vi "Pose3d_New.vi"(8 "Rotation3d":T1={"Q_quaternion"={"R"=1.0, "V"=[0.0, 0.0, 0.0]}}, 9 "z":dbl, 10 "Y":dbl, 11 "X":dbl) -> (3 "out Pose3d":T3={"Translation3d"={"X"=0.0, "Y"=0.0, "Z"=0.0}, "Rotation3d"={"Q_quaternion"={"R"=1.0, "V"=[0.0, 0.0, 0.0]}}} {"Translation3d"."Z" format="%14.3f"; "Translation3d"."Y" format="%14.3f"; "Translation3d"."X" format="%14.3f"})   [LabVIEW 2019, in "Trajectory_Library.lvlib"]
doc: "Constructs a pose with x, y, and z translations instead of a separate Translation3d.\n\nParameters:\n - X- The x component of the translational component of the pose.\n - Y - The y component of the translational component of the pose.\n - Z - The z component of the translational component of the pose.\n - Rotation3d - The rotational component of the pose.\n\nReturns:\n - OUT POSE3D - Output POSE3D"
uses:
  Trajectory_Library.lvlib
  TypeDef/QUATERNION.ctl
  TypeDef/ROTATION3D.ctl
  TypeDef/TRANSLATION3D.ctl
  POSE3D.ctl
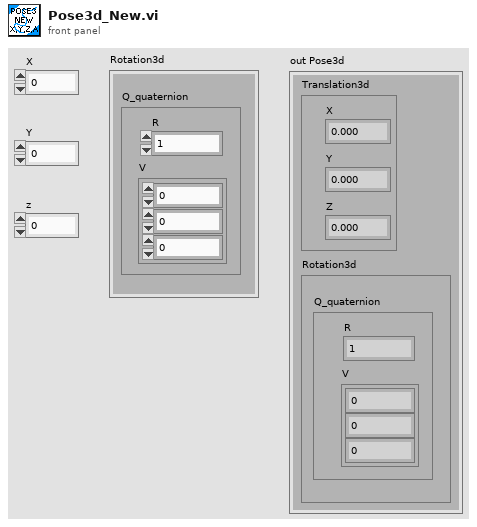
[diagram p1: front panel]
types:
  T1 = typedef "Trajectory_Library.lvlib/ROTATION3D.ctl" = cluster{"Q_quaternion":T2}
  T2 = typedef "Trajectory_Library.lvlib/QUATERNION.ctl" = cluster{"R":dbl, "V":dbl[]}
  T3 = typedef "Trajectory_Library.lvlib/POSE3D.ctl" = cluster{"Translation3d":T4, "Rotation3d":T1}
  T4 = typedef "Trajectory_Library.lvlib/TRANSLATION3D.ctl" = cluster{"X":dbl, "Y":dbl, "Z":dbl}
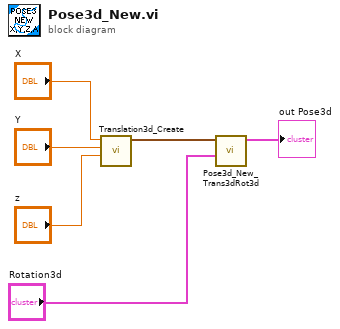
[diagram p0: block diagram]
diagram:
  n1 = call "Translation3d_Create.vi"("Z"="z", "Y"="Y", "X"="X") -> ("TRANSLATION3D"=w3:T4)  [unwired: 8 in]
  n2 = call "Pose3d_New_Trans3dRot3d.vi"("Rotation3d"="Rotation3d", "Translation3d"=w3) -> ("outPose3d"=→"out Pose3d":T3)  [unwired: 9 in]
